vi "Has Role.vi"(7 "Default if Blank (T)":bool=TRUE, 8 "error in (no error)":errorcluster, 10 "Role":string, 11 "Roles API in":refnum<class "Roles API.lvclass">) -> (0 "error out":errorcluster, 2 "Has Role":bool, 3 "Roles API out":refnum<class "Roles API.lvclass">)   [LabVIEW 2020, in "Volatus.lvlib" / "Roles API.lvclass"]
uses:
  Roles API.lvclass
  Roles API.lvclass/Roles API.ctl
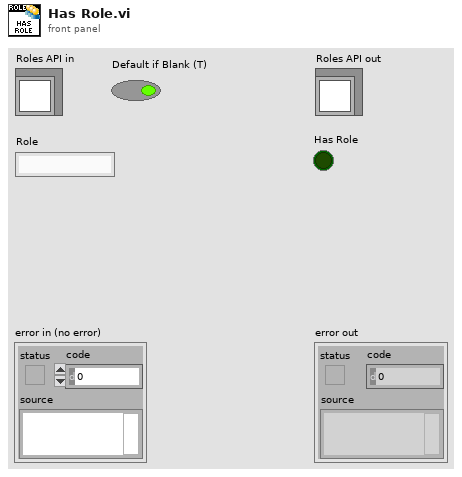
[diagram p1: front panel]
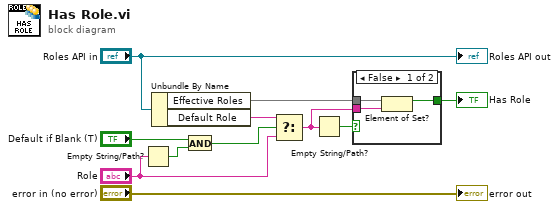
[diagram p0: block diagram]
diagram:
  n1 = Empty String/Path?(string/path="Role") -> (empty?=w6:bool)
  n2 = Unbundle By Name("Roles API in") -> ("Effective Roles"=w9:set{string}, "Default Role"=w5:string)
  n3 = And(x="Default if Blank (T)", y=w6) -> (x .and. y?=w3:bool)
  n4 = Select(t=w5, s=w3, f="Role") -> (s? t:f=w2:string)
  n5 = Empty String/Path?(string/path=w2) -> (empty?=w1:bool)
  n6 = case shown="False" w1 {
    selector: w1 -> [_ w15]
    tunnel: w9 -> [w14 _]
    tunnel: [w13 w15] -> w8
    tunnel: w2 -> [w12 _]
    frame False {
      n7 = Element of Set?(10:w12, 11:w14) -> (3:w13:bool)
    }
    frame True {
    }
  }
  "Has Role" <- w8
  "error out" <- "error in (no error)"
  "Roles API out" <- "Roles API in"
